vi "main.vi"() -> ()   [LabVIEW 2020]
uses:
  subVI/MsgBox.vi
  VarGLO/Global PEAK.vi
  <vilib>/regexp/Match Regular Expression.xnode
  VarGLO/Global var.vi
  VarGLO/VG_progressBar.vi
  f93c6fe3-7432-4718-be07-8f34c047d79f.vi
  VarGLO/Global PREDCIR.vi
  VarGLO/Global POSTDCIR.vi
  VarGLO/Global INTRADCIR.vi
  subVI/Ctrl/L2T.ctl
  <userlib>/Sylvain.lib/SN_type.ctl
panel:
  in  "TL?":bool
  in  "TypeVDA":T1
  out "POSTDCIR":T2
  out "PREDCIR":T2
  in  "40:2$ ok?":bool
  out "RunDCIR":bool
  out "INTRADCIR":T2
  out "dcir":string
  out "postdcir":string
  out "Numeric":i32 format="%.0f %"
  out "SNDCIR":string
  out "error out 2":errorcluster
  out "DCIR":u8(slide) scale=0.0..100.0
  in  "OFGETSVP$R":bool
  in  "stopask":bool
  in  "visadebug":refnum<visa-resource-name>
  out "String":string
  out "toute l'expression":string
  out "chaîne concaténée":string
  in  "image":string
  out "errout":errorcluster caption="sortie d'erreur"
  out "Image 2D":picture
  out "OFEnC":string caption="OF en cours coté Automate"
  out "err2":errorcluster
  out "MB":string
  in  "ValOFNext":bool
  in  "ok dem":bool
  in  "ValOF":bool
  out "intrafinal":string
  out "tableau ajouté":bool[](array[boolean])
  out "données":string[](array[string])
  out "OCV":string
  out "iso-":string
  out "iso+":string
  out "acir":string
  out "run..":i32(slide) scale=0.0..1000.0
  out "PN":string
  out "étage":string
  out "debug":T3
  in  "SimAuto":string caption="Simulateur automate"
  out "Check Final":bool
  out "mouchard OCV":string
  out "error out":errorcluster caption="Message erreur"
  in  "EXIT":bool
  out "L2T":T4 caption="Limites de test pris en compte"
  in  "OFnext":string caption="OF que l'on souhaite faire"
  out "STOP":bool
  out "Wdog":bool
  # "V3.3.0"
  # "Hors production\nZone de mise au point logiciel"
  # "Hors production\nZone de mise au point logiciel"
  # "--  Mouchard vers Auto  --"
  # "Test de mise au point"
  # "Pre DCIR_____________________________________"
  # "intra DCIR_____________________________________"
  # "Post DCIR_____________________________________"
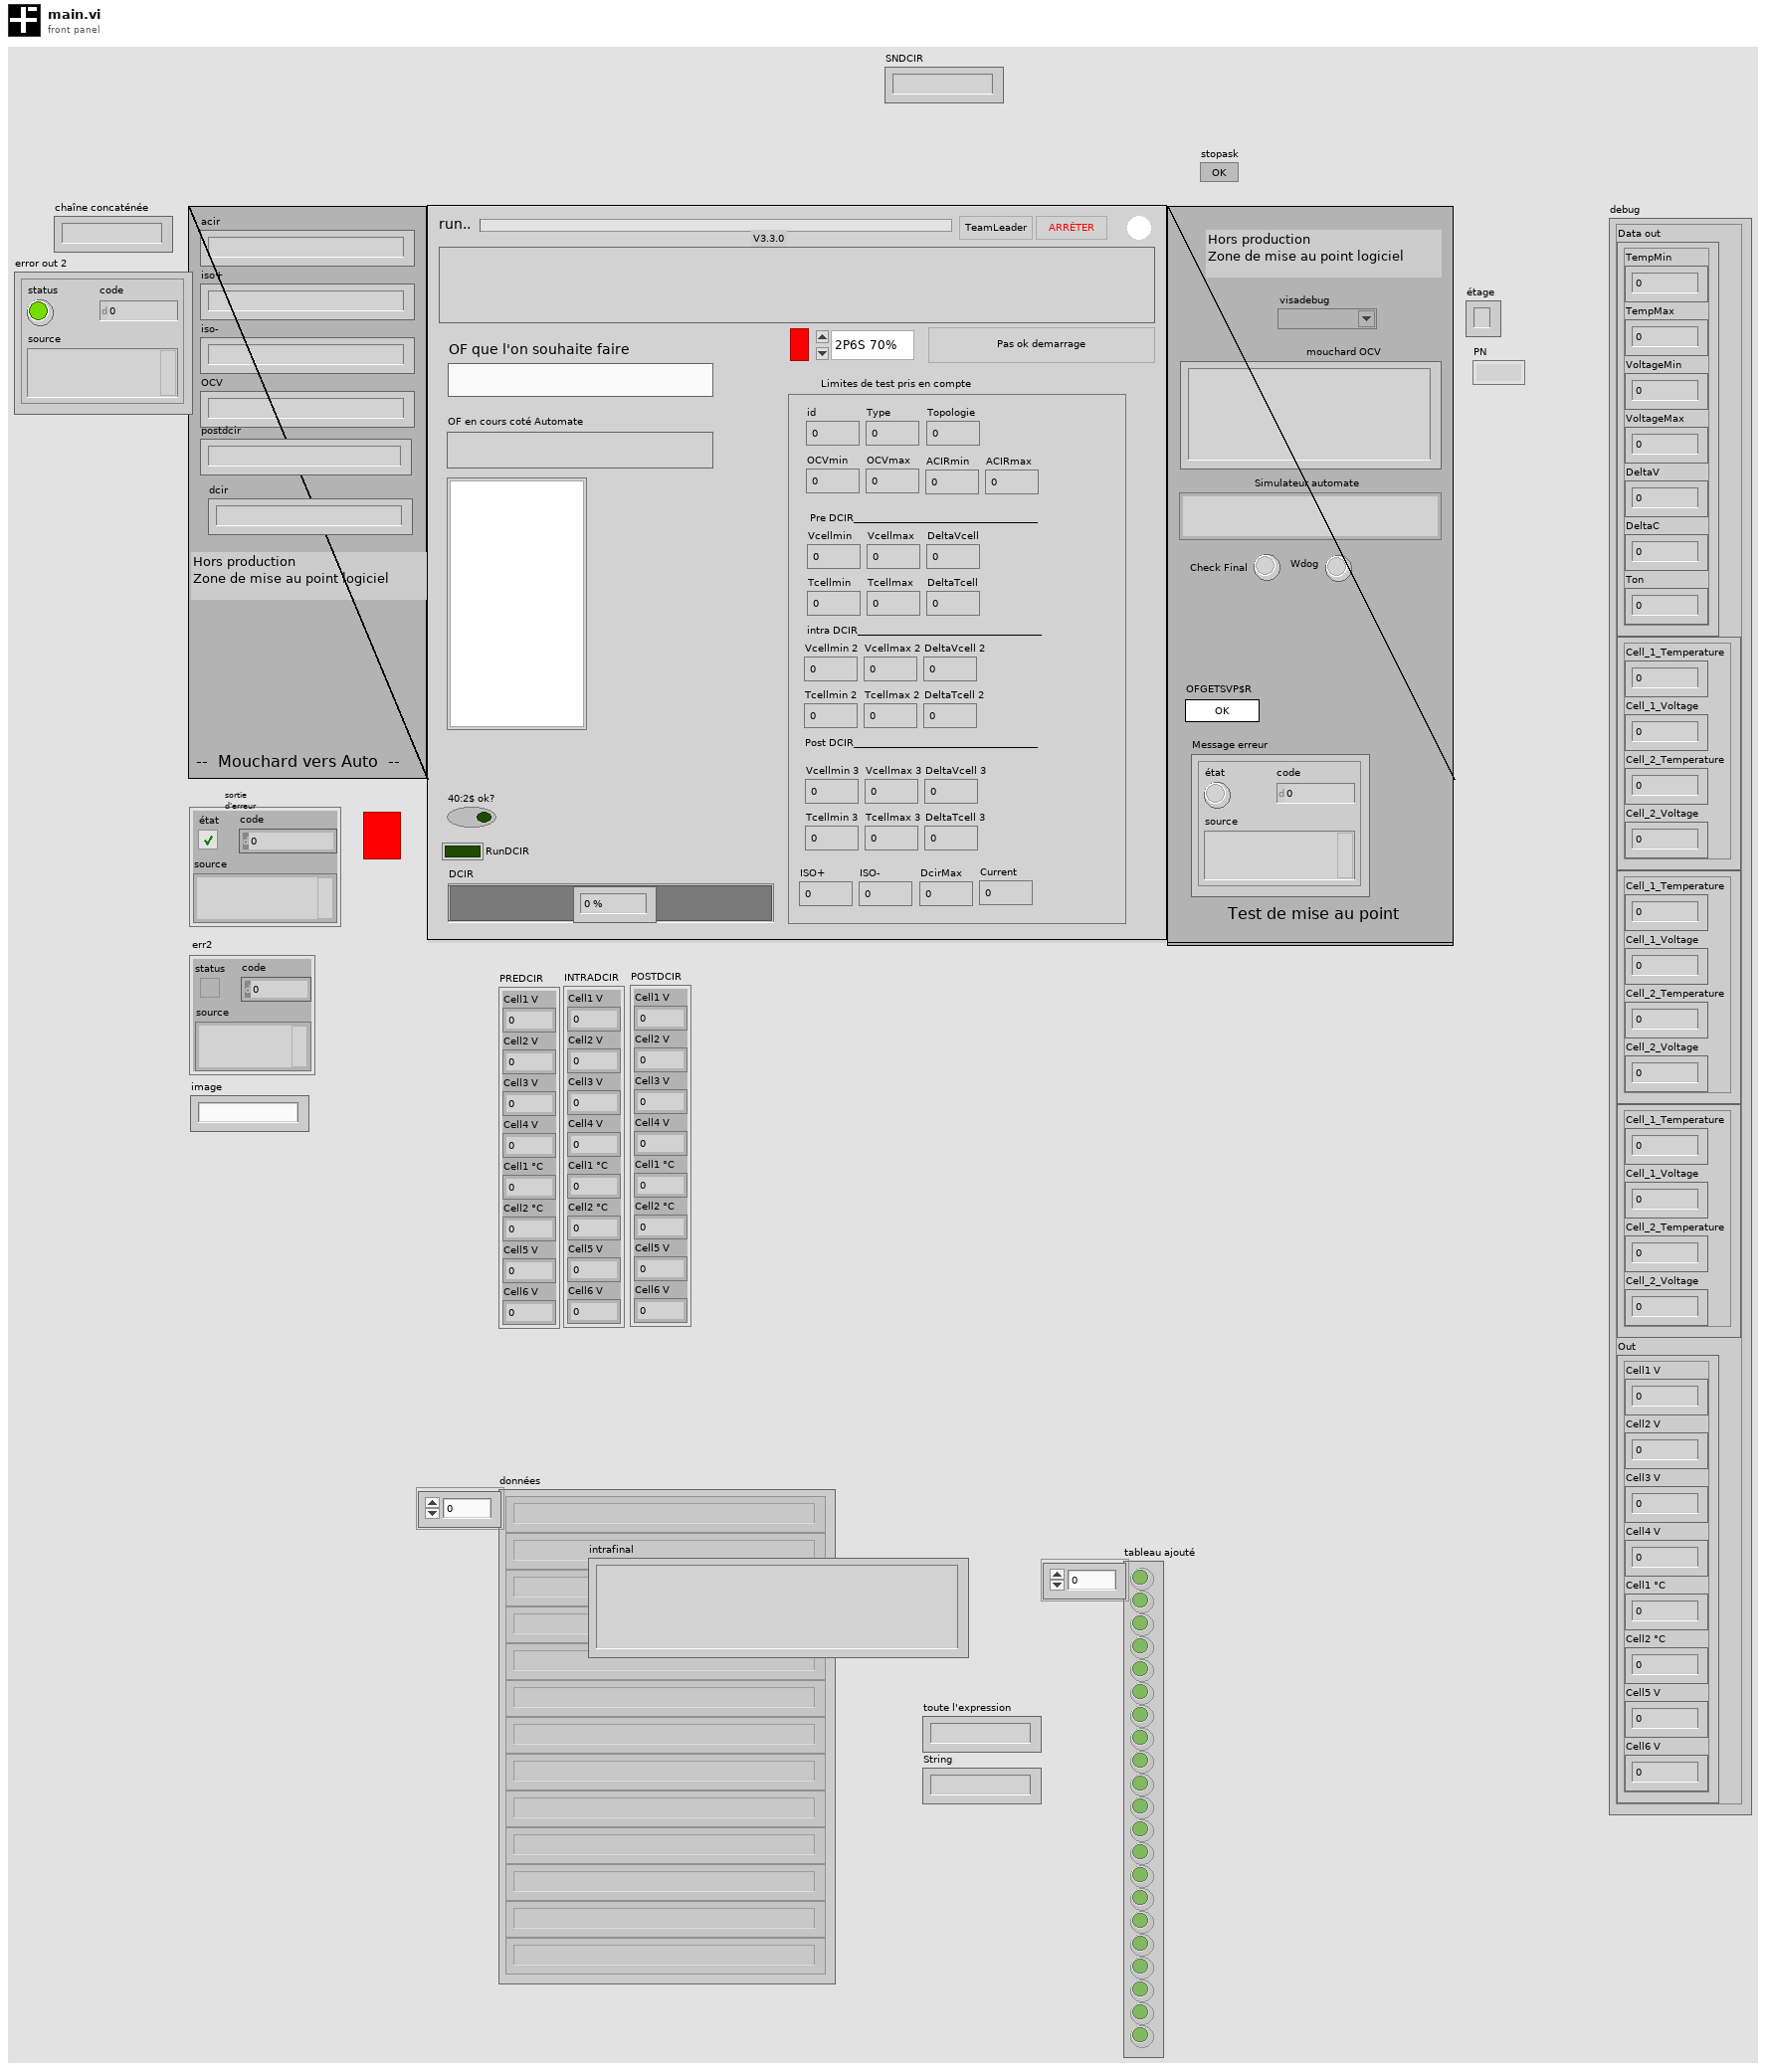
[diagram p1: front panel]
types:
  T1 = typedef "SN_type.ctl" = enum16{"2P6S 70%", "2P6S 30%", "3P4S 70%", "3P4S 30%"}
  T2 = cluster{"Cell1 V":sgl, "Cell2 V":sgl, "Cell3 V":sgl, "Cell4 V":sgl, "Cell1 °C":sgl, "Cell2 °C":sgl, "Cell5 V":sgl, "Cell6 V":sgl}
  T3 = cluster{"Data out":cluster{"TempMin":sgl, "TempMax":sgl, "VoltageMin":sgl, "VoltageMax":sgl, "DeltaV":sgl, "DeltaC":sgl, "Ton":sgl}, "Cluster":cluster{"Cell_1_Temperature":sgl, "Cell_1_Voltage":sgl, "Cell_2_Temperature":sgl, "Cell_2_Voltage":sgl}, "Cluster":cluster{"Cell_1_Temperature":sgl, "Cell_1_Voltage":sgl, "Cell_2_Temperature":sgl, "Cell_2_Voltage":sgl}, "Cluster":cluster{"Cell_1_Temperature":sgl, "Cell_1_Voltage":sgl, "Cell_2_Temperature":sgl, "Cell_2_Voltage":sgl}, "Out":cluster{"Cell1 V":sgl, "Cell2 V":sgl, "Cell3 V":sgl, "Cell4 V":sgl, "Cell1 °C":sgl, "Cell2 °C":sgl, "Cell5 V":sgl, "Cell6 V":sgl}}
  T4 = typedef "L2T.ctl" = cluster{"id":dbl, "Type":dbl, "OCVmin":dbl, "OCVmax":dbl, "ACIRmin":dbl, "ACIRmax":dbl, "Vcellmin":dbl, "Vcellmax":dbl, "DeltaVcell":dbl, "Tcellmin":dbl, "Tcellmax":dbl, "DeltaTcell":dbl, "ISO+":dbl, "ISO-":dbl, "DcirMax":dbl, "Current":dbl, "Topologie":dbl, "Vcellmin 2":dbl, "Vcellmax 2":dbl, "DeltaVcell 2":dbl, "Tcellmin 2":dbl, "Tcellmax 2":dbl, "DeltaTcell 2":dbl, "Vcellmin 3":dbl, "Vcellmax 3":dbl, "DeltaVcell 3":dbl, "Tcellmin 3":dbl, "Tcellmax 3":dbl, "DeltaTcell 3":dbl}
  T5 = cluster{"id":dbl, "Type":dbl, "OCVmin":dbl, "OCVmax":dbl, "ACIRmin":dbl, "ACIRmax":dbl, "Vcellmin":dbl, "Vcellmax":dbl, "DeltaVcell":dbl, "Tcellmin":dbl, "Tcellmax":dbl, "DeltaTcell":dbl, "ISO+":dbl, "ISO-":dbl, "DcirMax":dbl, "Current":dbl, "Topologie":dbl, "Vcellmin 2":dbl, "Vcellmax 2":dbl, "DeltaVcell 2":dbl, "Tcellmin 2":dbl, "Tcellmax 2":dbl, "DeltaTcell 2":dbl, "Vcellmin 3":dbl, "Vcellmax 3":dbl, "DeltaVcell 3":dbl, "Tcellmin 3":dbl, "Tcellmax 3":dbl, "DeltaTcell 3":dbl}
  T6 = typedef "PCANBasic.lvlib/Channel.ctl" = enum16{"PCAN_NONEBUS", "not used1", "not used2", "not used3", "not used4", "not used5", "not used6", "not used7", "not used8", "not used9", "not used10", "not used11", "not used12", "not used13", "not used14", "not used15", "not used16", "not used17", "not used18", "not used19", "not used20", "not used21", "not used22", "not used23", "not used24", "not used25", "not used26", "not used27", "not used28", "not used29", "not used30", "not used31", "not used32", "PCAN_ISABUS1", "PCAN_ISABUS2", "PCAN_ISABUS3", "PCAN_ISABUS4", "PCAN_ISABUS5", "PCAN_ISABUS6", "PCAN_ISABUS7", "PCAN_ISABUS8", "not used41", "not used42", "not used43", "not used44", "not used45", "not used46", "not used47", "not used48", "PCAN_DNGBUS1", "not used50", "not used51", "not used52", "not used53", "not used54", "not used55", "not used56", "not used57", "not used58", "not used59", "not used60", "not used61", "not used62", "not used63", "not used64", "PCAN_PCIBUS1", "PCAN_PCIBUS2", "PCAN_PCIBUS3", "PCAN_PCIBUS4", "PCAN_PCIBUS5", "PCAN_PCIBUS6", "PCAN_PCIBUS7", "PCAN_PCIBUS8", "not used73", "not used74", "not used75", "not used76", "not used77", "not used78", "not used79", "not used80", "PCAN_USBBUS1", "PCAN_USBBUS2", "PCAN_USBBUS3", "PCAN_USBBUS4", "PCAN_USBBUS5", "PCAN_USBBUS6", "PCAN_USBBUS7", "PCAN_USBBUS8", "Not used89", "Not used90", "Not used91", "Not used92", "Not used93", "Not used94", "Not used95", "Not used96", "PCAN_PCCBUS1", "PCAN_PCCBUS2"}
  T7 = typedef "imagedata.ctl" = cluster{"image type":i32, "image depth":i32, "image":u8[], "mask":u8[], "colors":u32[], "Rectangle":cluster{"left":i16, "top":i16, "right":i16, "bottom":i16}}
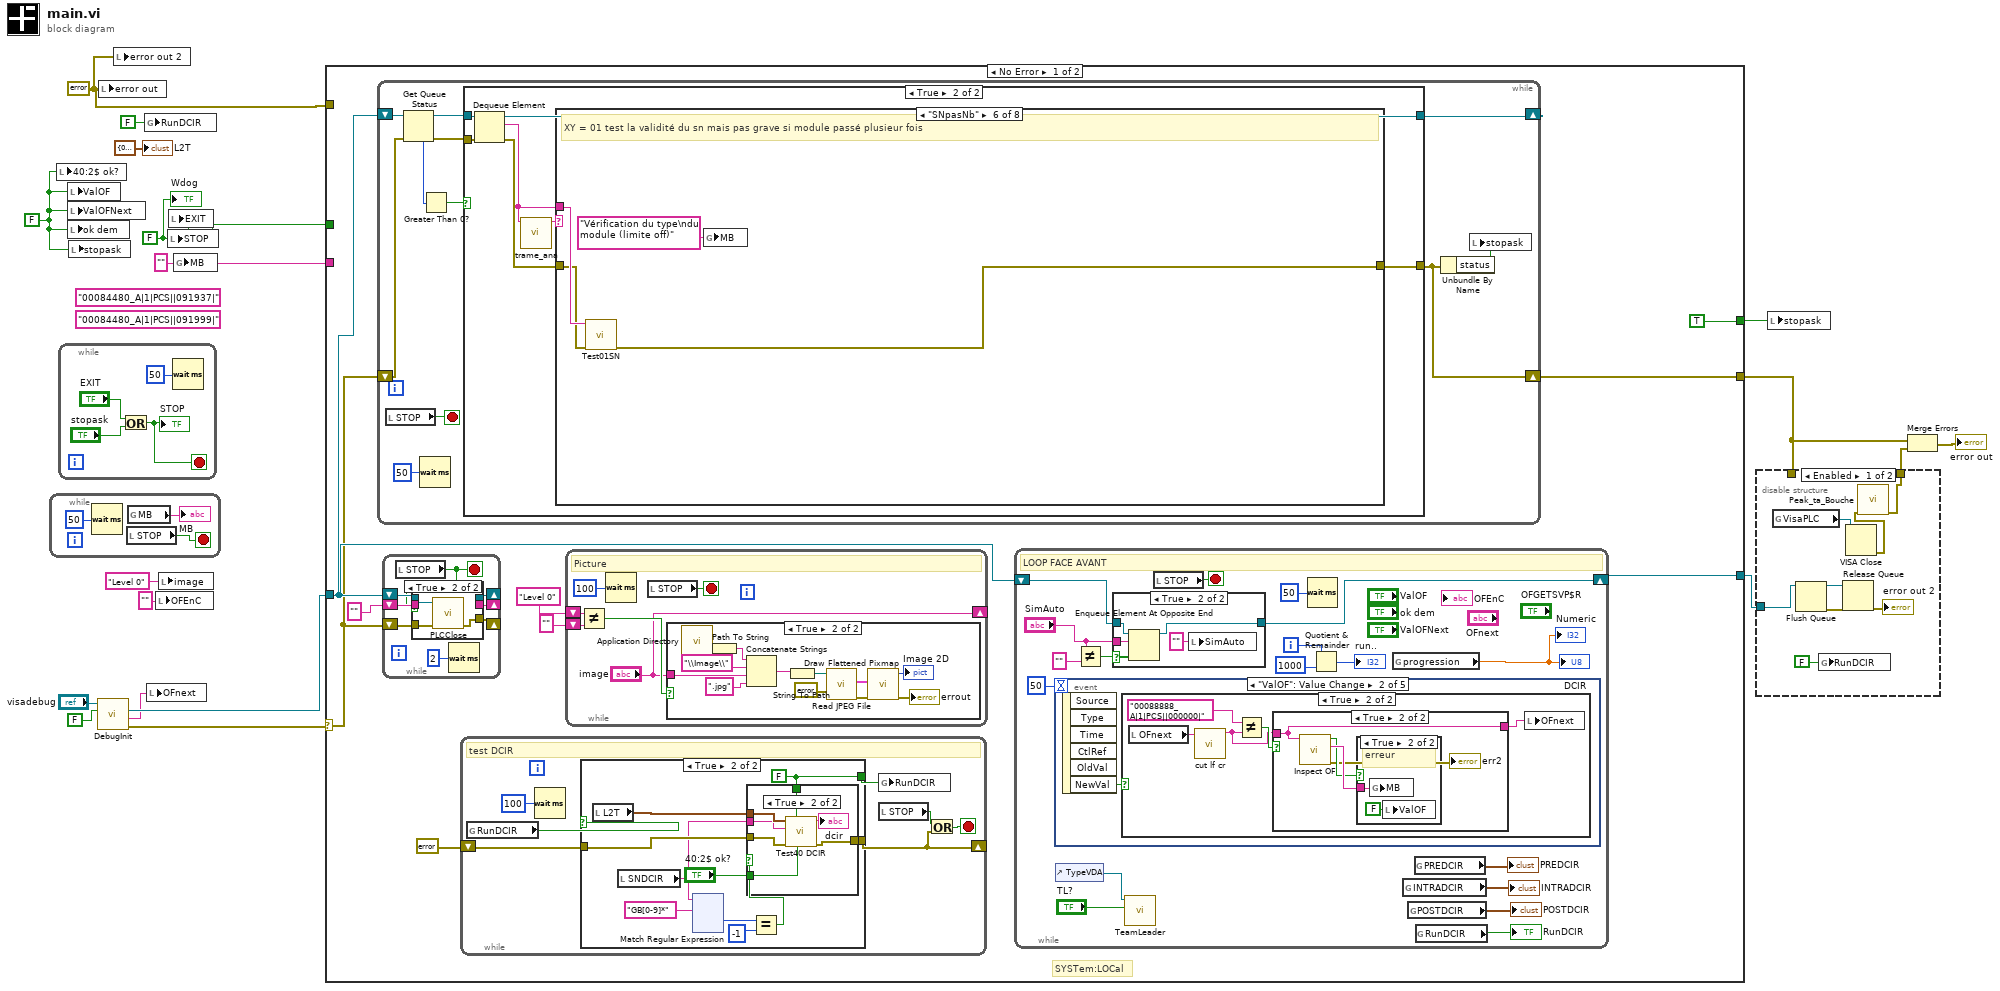
[diagram p0: block diagram]
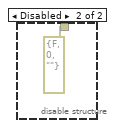
[diagram p2: hidden frame]
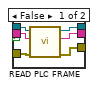
[diagram p3: hidden frame]
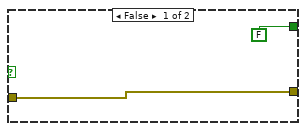
[diagram p4: hidden frame]
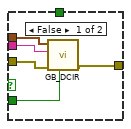
[diagram p5: hidden frame]
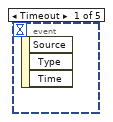
[diagram p6: hidden frame]
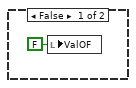
[diagram p7: hidden frame]
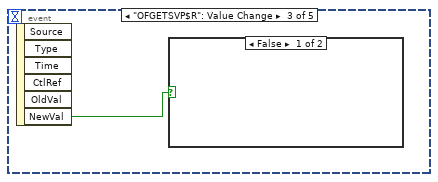
[diagram p10: hidden frame]
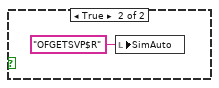
[diagram p11: hidden frame]
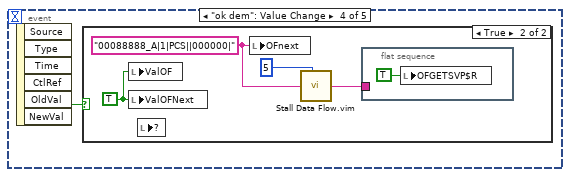
[diagram p12: hidden frame]
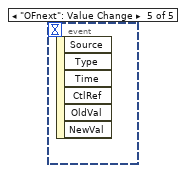
[diagram p14: hidden frame]
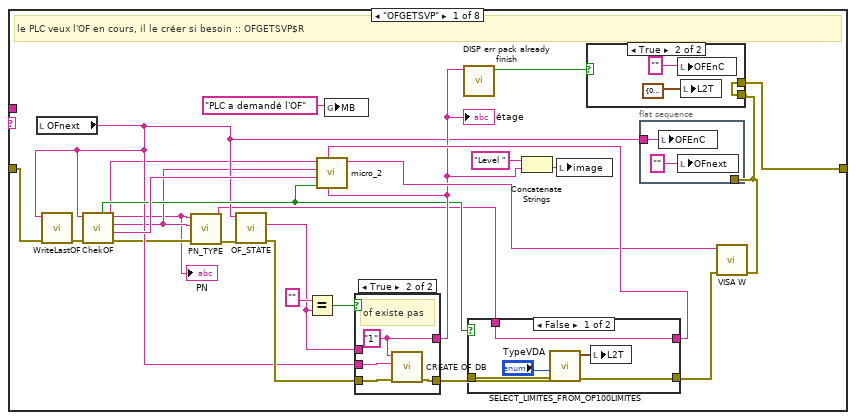
[diagram p17: hidden frame]
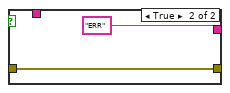
[diagram p20: hidden frame]
diagram:
  w1 = FALSE ("OF OK démarrage")
  w2 = errorcluster {"status"=FALSE, "code"=0, "source"=""} ("error out")
  (unwired) "00084480_A|1|PCS||091999|" ("OF à faire après")
  (unwired) "00084480_A|1|PCS||091937|" ("OF à faire")
  w14 = "" ("MSG")
  w18 = FALSE ("Tickwatchdog")
  n1 = while {
    stop <- w20 stop-if-true
    n2 = Wait (ms) ("Attendre (ms)")(milliseconds to wait=u32 50 ("attente (ms)")) -> ()  [unwired: 1 out]
    n3 = local read "STOP"() -> (w20:bool)
    n4 = global read "MsgBox.vi" "MB"() -> (→"MB":string)
  }
  n5 = local write "40:2$ ok?"(w1) -> ()
  n6 = while {
    stop <- w22 stop-if-true
    n7 = Or(x="EXIT", y="stopask") -> (x .or. y?=w22:bool)
    "STOP" <- w22
    n8 = Wait (ms)(milliseconds to wait=u32 50) -> ()  [unwired: 1 out]
  }
  n9 = local write "ValOF"(w1) -> ()
  n10 = local write "ValOFNext"(w1) -> ()
  n11 = local write "ok dem"(w1) -> ()
  n12 = local write "stopask"(w1) -> ()
  n13 = call "DebugInit.vi"("debug?"=FALSE ("s"), "VISA Refnum in"="visadebug") -> ("error out"=w10:errorcluster, "OF"=w11:string, "queue out"=w17:refnum<queue>)  [unwired: 7 in]
  n14 = local write "error out"(w2) -> ()
  n15 = local write "error out 2"(w2) -> ()
  n16 = global write "Global var.vi" "RunDCIR"(FALSE ("RunDCIR")) -> ()
  n17 = local write "OFnext"(w11) -> ()
  n18 = local write "OFEnC"("" ("OFEnC")) -> ()
  n19 = local write "image"("Level 0" ("image")) -> ()
  n20 = local write "STOP"(w18) -> ()
  n21 = local write "EXIT"(w18) -> ()
  n22 = global write "MsgBox.vi" "MB"(w14) -> ()
  n23 = case shown="No Error" w10 {
    selector: w10 -> [w29 w541]
    tunnel: w18 -> [_ _]
    tunnel: w14 -> [_ _]
    tunnel: w17 -> [w33 w539]
    tunnel: w2 -> [_ w544]
    tunnel: [w32 w544] -> w7
    tunnel: [TRUE TRUE] -> w5
    tunnel: [w27 w539] -> w4
    frame No Error {
      # "SYSTem:LOCal"
      n24 = while {
        shift-right: [w244] -> w32
        shift-left: w29 -> [w252]
        shift-right: [w248] -> _
        shift-left: w33 -> [w251]
        stop <- w246 stop-if-true
        n25 = local read "STOP"() -> (w246:bool)
        n26 = Get Queue Status ("Obtenir l'état d'une file d'attente")(queue=w251, error in (no error)=w252) -> (queue out=w250:refnum<queue>, error out=w249:errorcluster, # elements in queue=w245:i32)  [unwired: 1 in, 5 out]
        n27 = Wait (ms) ("Attendre (ms)")(milliseconds to wait=u32 50 ("attente (ms)")) -> ()  [unwired: 1 out]
        n28 = Greater Than 0?(x=w245) -> (x > 0?=w247:bool)
        n29 = case shown="True" w247 {
          tunnel: w250 -> [w253 w260]
          tunnel: w249 -> [w254 w259]
          tunnel: [w254 w257] -> w244
          tunnel: [w253 w256] -> w248
          frame False {
          }
          frame True {
            n30 = Dequeue Element(queue=w260, error in (no error)=w259) -> (queue out=w256:refnum<queue>, element=w255:string, error out=w258:errorcluster)  [unwired: 1 in, 1 out]
            n31 = call "trame_ana.vi"("Chaîne"=w255) -> ("Instruction"=w261:string)  [unwired: 10 in]
            n32 = case shown="\"SNpasNb\"" w261 {
              tunnel: w258 -> [w279 w309 w322 w495 w504 w512 w515 w520]
              tunnel: [w271 w308 w323 w494 w499 w514 w517 w520] -> w257
              tunnel: w255 -> [_ w312 w318 w492 w503 w513 w516 w519]
              frame "OFGETSVP" {
                # "le PLC veux l'OF en cours, il le créer si besoin :: OFGETSVP$R"
                n33 = local read "OFnext"() -> (w267:string)
                n34 = call "WriteLastOF.vi"("errin"=w279, "OF to save"=w267) -> ("errout"=w278:errorcluster)  [unwired: 9 in]
                n35 = call "ChekOF.vi"("errin"=w278, "OF in"=w267) -> ("errout"=w266:errorcluster, "SN"=w286:string, "version"=w265:string, "PN"=w264:string, "ArrsurErr"=w270:bool)  [unwired: 4 in, 1 out]
                "PN" <- w264
                n36 = call <userlib>:"PN_TYPE.vi"("errin"=w266, "Variante"=w265, "PN"=w264) -> ("errout"=w263:errorcluster, "element"=w262:string)  [unwired: 7 in]
                n37 = call <userlib>:"OF_STATE.vi"("errin"=w263, "OF"=w267) -> ("error out"=w269:errorcluster, "state str"=w268:string)  [unwired: 6 in, 2 out]
                n38 = Equal? ("Égaux ?")(x="", y=w268) -> (x = y?=w285:bool)
                n39 = global write "MsgBox.vi" "MB"("PLC a demandé l'OF" ("MSG")) -> ()
                n40 = case shown="True" w285 {
                  tunnel: w269 -> [w293 w298]
                  tunnel: w267 -> [_ w297]
                  tunnel: [w294 w296] -> w274
                  tunnel: w268 -> [w294 _]
                  tunnel: [w293 w295] -> w284
                  frame False {
                  }
                  frame True {
                    w296 = "1" ("result")
                    # "of existe pas"
                    n41 = call "CREATE OF DB.vi"("errin"=w298, "OF"=w297, "state"=w296) -> ("error out"=w295:errorcluster)  [unwired: 8 in]
                  }
                }
                "étage" <- w274
                n42 = call "DISP err pack already finish.vi"("result"=w274) -> ("étage3"=w273:bool)  [unwired: 10 in]
                n43 = case shown="False" w270 {
                  tunnel: [w303 w304] -> w283
                  tunnel: [w300 "ERR" ("Type")] -> w282
                  tunnel: w284 -> [w302 w304]
                  tunnel: w262 -> [w300 _]
                  frame False {
                    n44 = call <userlib>:"SELECT_LIMITES_FROM_OP100LIMITES.vi"("errin"=w302, "Enum"="TypeVDA") -> ("errout"=w303:errorcluster, "data"=w301:T4)  [unwired: 7 in, 1 out]
                    n45 = local write "L2T"(w301) -> ()
                  }
                  frame True {
                  }
                }
                n46 = call "micro_2.vi"("result"=w274, "Type"=w282, "err"=w270, "SN"=w286, "version"=w265, "PN"=w264) -> ("Chaîne"=w281:string)  [unwired: 5 in]
                n47 = Concatenate Strings("Level " ("string"), w274) -> (w275:string)
                n48 = local write "image"(w275) -> ()
                n49 = flat-sequence {
                  tunnel: w267 -> [w292]
                  tunnel: w272 -> [_]
                  frame #0 {
                    n50 = local write "OFEnC"(w292) -> ()
                    n51 = local write "OFnext"("" ("OFnext")) -> ()
                  }
                }
                n52 = call "VISA W.vi"("errin"=w283, "Chaîne"=w281) -> ("errout"=w272:errorcluster)  [unwired: 9 in]
                n53 = case shown="True" w273 {
                  tunnel: w272 -> [w287 w289]
                  tunnel: [w287 w289] -> w271
                  frame False {
                  }
                  frame True {
                    n54 = local write "OFEnC"("" ("OFEnC")) -> ()
                    n55 = local write "L2T"(T5 {"id"=0.0, "Type"=0.0, "OCVmin"=0.0, "OCVmax"=0.0, "ACIRmin"=0.0, "ACIRmax"=0.0, "Vcellmin"=0.0, "Vcellmax"=0.0, "DeltaVcell"=0.0, "Tcellmin"=0.0, "Tcellmax"=0.0, "DeltaTcell"=0.0, "ISO+"=0.0, "ISO-"=0.0, "DcirMax"=0.0, "Current"=0.0, "Topologie"=0.0, "Vcellmin 2"=0.0, "Vcellmax 2"=0.0, "DeltaVcell 2"=0.0, "Tcellmin 2"=0.0, "Tcellmax 2"=0.0, "DeltaTcell 2"=0.0, "Vcellmin 3"=0.0, "Vcellmax 3"=0.0, "DeltaVcell 3"=0.0, "Tcellmin 3"=0.0, "Tcellmax 3"=0.0, "DeltaTcell 3"=0.0} ("L2T")) -> ()
                  }
                }
              }
              frame "OFFINISH" {
                # "OFFINISHOK200084480_A|1|PCS||00001|$R"
                # "\" OFFINISHOK200084480_A|1|PCS||00001|$R \""
                n56 = local read "OFEnC"() -> (w310:string)
                n57 = local read "étage"() -> (w311:string)
                n58 = call "OFFINISH_compare.vi"("errin"=w309, "PlcFrame"=w312, "étage"=w311, "OFenC"=w310) -> ("errout"=w308:errorcluster, "OFEnC"=w306:string, "L2T"=w307:T5, "MB"=w313:string)  [unwired: 4 in]
                n59 = local write "OFEnC"(w306) -> ()
                n60 = global write "MsgBox.vi" "MB"(w313) -> ()
                n61 = local write "L2T"(w307) -> ()
              }
              frame "Requette" {
                # "SN"
                n62 = String Subset ("Sous-ensemble d'une chaîne")(string=w318, length (rest)=2 ("longueur (reste)")) -> (substring=w324:string)  [unwired: 1 in]
                n63 = xnode "Match Regular Expression"("chaîne en entrée"=w318, "expression régulière"="[0-9 A-Z]*:", "offset (0)"=2) -> ("toute l'expression"=w317:string, "après la correspondance"=w321:string)  [unwired: 3 in, 3 out]
                n64 = Search and Replace String ("Rechercher et remplacer une chaîne")(input string=w321, search string="$R" ("chaîne recherchée")) -> (result string=w319:string)  [unwired: 6 in, 3 out]
                n65 = Search and Replace String(input string=w317, search string=":", replace string="" ("replace string (\"\")")) -> (result string=w314:string)  [unwired: 5 in, 3 out]
                n66 = case shown="\"50\"" w324 {
                  tunnel: [w329 w339 w346 w352 w358 w364 w371] -> w323
                  tunnel: w322 -> [w329 w340 w343 w349 w355 w364 w373]
                  tunnel: w319 -> [_ w338 w347 w353 w361 _ _]
                  tunnel: w314 -> [_ w336 w345 w351 w360 w362 w370]
                  frame "Faux", Default {
                    n67 = global write "MsgBox.vi" "MB"("J'ai recu une trame non comprise" ("MSG")) -> ()
                  }
                  frame "10" {
                    w337 = "!!!!!" ("chaîne")
                    # "OCV ( PLC ) + CMODpredcir( PC )"
                    n68 = local read "L2T"() -> (w330:T4)
                    n69 = global read "Global PEAK.vi" "T10"() -> (w331:T6)
                    n70 = global write "MsgBox.vi" "MB"("PLC demande à verifier\nl'OCV" ("MSG")) -> ()
                    n71 = call "Test10.vi"("Peak"=w331, "L2T"=w330, "errin"=w340, "SN"=w336, "OCV"=w338) -> ("errout"=w339:errorcluster, "chaîne concaténée"=w335:string, "cluster de sortie"=→"debug":T3)  [unwired: 3 in, 1 out]
                    n72 = Concatenate Strings(w338, w337, w336, w337, w335) -> (→"mouchard OCV":string)
                  }
                  frame "11" {
                    # "ACIR :: PLC"
                    n73 = local read "L2T"() -> (w341:T4)
                    n74 = call "Test11ACiR.vi"("errin"=w343, "L2T 2"=w341, "result string"=w347, "SN"=w345) -> ("error out"=w346:errorcluster, "String"=→"acir":string)  [unwired: 6 in]
                    n75 = global write "MsgBox.vi" "MB"("Le PLC demande à verifier \nl'ACIR" ("MSG")) -> ()
                  }
                  frame "20" {
                    # "ISOLEMENT BAT + :: PLC"
                    n76 = local read "L2T"() -> (w354:T4)
                    n77 = call "Test20ISO+.vi"("errin"=w349, "L2T 2"=w354, "mesure"=w353, "SN"=w351) -> ("error out"=w352:errorcluster, "iso+"=→"iso+":string)  [unwired: 6 in]
                    n78 = global write "MsgBox.vi" "MB"("Le PLC veux vérifier\nl'isolement BAT+" ("MSG")) -> ()
                  }
                  frame "30" {
                    # "ISOLEMENT BAT -  :: PLC"
                    n79 = local read "L2T"() -> (w359:T4)
                    n80 = call "Test30ISOmoins.vi"("errin"=w355, "L2T"=w359, "Value"=w361, "SN"=w360) -> ("error out"=w358:errorcluster, "ISO-"=→"iso-":string)  [unwired: 6 in]
                    n81 = global write "MsgBox.vi" "MB"("Le PLC veux vérifier\nl'isolement BAT-" ("MSG")) -> ()
                  }
                  frame "40" {
                    # "400B5MEVA000CA1JC1M5525088:0$R"
                    # "DCIR :: PC"
                    n82 = global write "Global var.vi" "RunDCIR"(TRUE) -> ()
                    n83 = global write "MsgBox.vi" "MB"("PLC demande un DCIR" ("MSG")) -> ()
                    "SNDCIR" <- w362
                  }
                  frame "50" {
                    # "post DCIR :: PC"
                    n84 = global read "Global PEAK.vi" "T50"() -> (w374:T6)
                    n85 = local read "L2T"() -> (w367:T4)
                    n86 = call "Test50.vi"("L2T"=w367, "SN"=w370, "errin"=w373, "Peak"=w374) -> ("v1"=→"postdcir":string, "errout"=w372:errorcluster)  [unwired: 4 in, 1 out]
                    n87 = call "FinalCheck.vi"("errin"=w372, "L2T"=w367, "SN"=w370) -> ("error out"=w371:errorcluster, "ET logique"=→"Check Final":bool)  [unwired: 4 in, 3 out]
                    n88 = global write "MsgBox.vi" "MB"("PLC demande un Post DCIR" ("MSG")) -> ()
                  }
                }
              }
              frame "TracaHIOKI" {
                # "INSERT INTO `zen+`.`op100eqsn` (`id`, `PNvers`, `etageencours`, `snst5520isoplus`\n, `snst5520isomoins`, `snbt3563`, `date`) VALUES ('3', 'OFIII', '2', 'iso+', 'iso-', '35', '2023-06-06 23:55:33');"
                n89 = local read "étage"() -> (w491:string)
                n90 = local read "PN"() -> (w490:string)
                n91 = call "TracaHioki.vi"("errin"=w495, "datain"=w492, "etage"=w491, "PN"=w490) -> ("error out"=w494:errorcluster, "out"=w493:string)  [unwired: 6 in]
                n92 = local write "mouchard OCV"(w493) -> ()
                n93 = global write "MsgBox.vi" "MB"("Je releve le SN du ST5520 Iso+" ("Message BOX")) -> ()
              }
              frame "SN" {
                # "XY = 00 test la validité du SN"
                n94 = local read "L2T"() -> (w496:T4)
                n95 = call "Test00SN.vi"("errin"=w504, "L2T 2"=w496, "String in"=w503) -> ("errout"=w500:errorcluster, "toute l'expression"=w502:string, "Boolean"=w498:bool, "String out"=w501:string)  [unwired: 5 in]
                n96 = case shown="True" w498 {
                  tunnel: w502 -> [_ w510]
                  tunnel: w501 -> [_ w509]
                  tunnel: w500 -> [w505 w508]
                  tunnel: [w505 w507] -> w499
                  frame False {
                  }
                  frame True {
                    n97 = call "Init Data BDD.vi"("errin"=w508, "Type"=w509, "SN"=w510) -> ("error out"=w507:errorcluster, "chaîne concaténée"=→"chaîne concaténée":string)  [unwired: 7 in]
                    "toute l'expression" <- w510
                    "String" <- w509
                  }
                }
                n98 = global write "MsgBox.vi" "MB"("Vérification du SN et du type\ndu module" ("Message BOX")) -> ()
              }
              frame "SNpasNb" {
                # "XY = 01 test la validité du sn mais pas grave si module passé plusieur fois"
                n99 = call "Test01SN.vi"("errin"=w512, "String"=w513) -> ("errout"=w514:errorcluster)  [unwired: 9 in]
                n100 = global write "MsgBox.vi" "MB"("Vérification du type\ndu module (limite off)" ("Message BOX")) -> ()
              }
              frame "GB" {
                # "Cas des Goldens boards Obsolète"
                n101 = call "TestGB.vi"("errin"=w515, "String"=w516) -> ("errout"=w517:errorcluster)  [unwired: 9 in]
                n102 = global write "MsgBox.vi" "MB"("Golden Board engagé" ("Message BOX")) -> ()
              }
              frame "ERR", Default {
                n103 = call "DISP err unknow request.vi"("String"=w519) -> ()  [unwired: 11 in]
              }
            }
          }
        }
        n104 = Unbundle By Name(w244) -> ("status"=w243:bool)
        n105 = local write "stopask"(w243) -> ()
      }
      n106 = while {
        shift-right: [w37] -> _
        shift-left: "" -> [w38]
        shift-right: [w39] -> _
        shift-left: w29 -> [w42]
        shift-right: [w40] -> _
        shift-left: w33 -> [w41]
        stop <- w36 stop-if-true
        n107 = local read "STOP"() -> (w36:bool)
        n108 = case shown="True" w36 {
          tunnel: w42 -> [w48 w51]
          tunnel: w41 -> [w47 w50]
          tunnel: [w46 _] -> w40
          tunnel: [w45 w49] -> w39
          tunnel: w38 -> [w44 _]
          tunnel: [w43 _] -> w37
          frame False {
            n109 = call "READ PLC FRAME.vi"("errin"=w48, "String in"=w44, "Queue in"=w47) -> ("errout"=w45:errorcluster, "String out"=w43:string, "Queue out"=w46:refnum<queue>)  [unwired: 6 in]
          }
          frame True {
            n110 = call "PLCClose.vi"("error in (no error)"=w51, "Queue in"=w50) -> ("error out"=w49:errorcluster)  [unwired: 9 in]
          }
        }
        n111 = Wait (ms)(milliseconds to wait=u32 2) -> ()  [unwired: 1 out]
      }
      n112 = while {
        shift-right: [w55] -> _
        shift-left: errorcluster {"status"=FALSE, "code"=0, "source"=""} ("errout") -> [w56]
        stop <- w53 stop-if-true
        # "test DCIR"
        n113 = global read "Global var.vi" "RunDCIR"() -> (w57:bool)
        n114 = Wait (ms) ("Attendre (ms)")(milliseconds to wait=u32 100 ("attente (ms)")) -> ()  [unwired: 1 out]
        n115 = case shown="True" w57 {
          tunnel: w56 -> [w60 w69]
          tunnel: [w60 w68] -> w55
          tunnel: [FALSE ("3P4S") w67] -> w52
          frame False {
          }
          frame True {
            w67 = FALSE ("3P4S")
            n116 = local read "L2T"() -> (w70:T4)
            n117 = local read "SNDCIR"() -> (w65:string)
            n118 = xnode "Match Regular Expression"("input string"=w65, "regular expression"="GB[0-9]*") -> ("offset past match"=w64:i32)  [unwired: 4 in, 4 out]
            n119 = Equal?(x=w64, y=-1) -> (x = y?=w62:bool)
            n120 = case shown="True" w62 {
              tunnel: w70 -> [w72 w82]
              tunnel: w69 -> [w74 w81]
              tunnel: [w75 w80] -> w68
              tunnel: w67 -> [_ w79]
              tunnel: w65 -> [w73 w78]
              tunnel: "40:2$ ok?" -> [w71 w76]
              frame False {
                n121 = call "GB_DCIR.vi"("40:2$ ok?"=w71, "errin"=w74, "SN"=w73, "L2T 2"=w72) -> ("errout"=w75:errorcluster)  [unwired: 7 in]
              }
              frame True {
                n122 = call "Test40 DCIR.vi"("40:2$ ok?"=w76, "3P4S"=w79, "errin"=w81, "SN"=w78, "L2T 2"=w82) -> ("errout"=w80:errorcluster, "v1"=→"dcir":string)  [unwired: 1 in, 4 out]
              }
            }
          }
        }
        n123 = global write "Global var.vi" "RunDCIR"(w52) -> ()
        n124 = local read "STOP"() -> (w54:bool)
        n125 = Or(x=w54, y=w55) -> (x .or. y?=w53:bool)
      }
      n126 = while {
        shift-right: ["image"] -> _
        shift-left: "" ("image") -> [w522]
        shift-left: "Level 0" ("image") -> [w521]
        stop <- w525 stop-if-true
        # "Picture"
        n127 = Not Equal?(x=w521, y=w522) -> (x != y?=w524:bool)
        n128 = Wait (ms) ("Attendre (ms)")(milliseconds to wait=u32 100 ("attente (ms)")) -> ()  [unwired: 1 out]
        n129 = local read "STOP"() -> (w525:bool)
        n130 = case shown="True" w524 {
          tunnel: "image" -> [_ w536]
          frame False {
          }
          frame True {
            n131 = call <vilib>:"Application Directory.vi"() -> ("Application Directory"=w532:path)
            n132 = Path To String(path=w532) -> (string=w533:string)
            n133 = Concatenate Strings(w533, "\\Image\\" ("chaîne"), w536, ".jpg" ("chaîne")) -> (w531:string)
            n134 = String To Path(string=w531) -> (path=w530:path)
            n135 = call <vilib>:"Read JPEG File.vi"("error in (no error)"=errorcluster {"status"=FALSE, "code"=0, "source"=""}, "path to JPEG file"=w530) -> ("error out"=→"errout":errorcluster, "image data"=w537:T7)  [unwired: 7 in, 1 out]
            n136 = call <vilib>:"Draw Flattened Pixmap.vi"("image data"=w537) -> ("new picture"=→"Image 2D":picture)  [unwired: 8 in]
          }
        }
      }
      n137 = while {
        shift-right: [w211] -> w27
        shift-left: w33 -> [w212]
        i -> [w205]
        stop <- w214 stop-if-true
        # "LOOP FACE AVANT"
        n138 = event shown="[1] \"ValOF\": Value Change" {
          selector: _ -> [_ _ _ _ _]
          dyn-events: _ -> [_ _ _ _ _]
          timeout: 50 -> [_ _ _ _ _]
          event Timeout {
            n139 = event-data() -> ()  [unwired: 1 in, 3 out]
          }
          event "ValOF": Value Change {
            n140 = event-data() -> ("NewVal"=w215:bool)  [unwired: 1 in, 5 out]
            n141 = case shown="True" w215 {
              frame False {
                n142 = local write "ValOF"(FALSE ("Bouton Jouer")) -> ()
              }
              frame True {
                n143 = local read "OFnext"() -> (w221:string)
                n144 = call "cut lf cr.vi"("strin"=w221) -> ("strout"=w217:string)  [unwired: 10 in]
                n145 = Not Equal?(x="00088888_A|1|PCS||000000|", y=w217) -> (x != y?=w219:bool)
                n146 = case shown="True" w219 {
                  tunnel: w217 -> [w222 w223]
                  tunnel: [w222 w223] -> w218
                  frame False {
                  }
                  frame True {
                    n147 = call "Inspect OF.vi"("OF"=w223) -> ("error out"=→"err2":errorcluster, "cas faux"=w226:string, "Boolean"=w225:bool)  [unwired: 8 in]
                    n148 = case shown="True" w225 {
                      tunnel: w226 -> [_ w227]
                      frame False {
                      }
                      frame True {
                        # "erreur"
                        n149 = global write "MsgBox.vi" "MB"(w227) -> ()
                        n150 = local write "ValOF"(FALSE ("Bouton Jouer")) -> ()
                      }
                    }
                  }
                }
                n151 = local write "OFnext"(w218) -> ()
              }
            }
          }
          event "OFGETSVP$R": Value Change {
            n152 = event-data() -> ("NewVal"=w229:bool)  [unwired: 1 in, 5 out]
            n153 = case shown="False" w229 {
              frame False {
              }
              frame True {
                n154 = local write "SimAuto"("OFGETSVP$R" ("SimAuto")) -> ()
              }
            }
          }
          event "ok dem": Value Change {
            n155 = event-data() -> ("NewVal"=w231:bool)  [unwired: 1 in, 5 out]
            n156 = case shown="True" w231 {
              frame False {
              }
              frame True {
                w235 = TRUE ("Bouton Jouer")
                w234 = "00088888_A|1|PCS||000000|" ("OF à faire")
                n157 = local write "ValOF"(w235) -> ()
                n158 = local write "ValOFNext"(w235) -> ()
                n159 = local read item#-1() -> ()  [unwired: 1 in]
                n160 = local write "OFnext"(w234) -> ()
                n161 = call "Stall Data Flow.vim"("value in"=w234, "milliseconds to wait"=u32 5) -> ("value out"=w233:string)  [unwired: 1 out]
                n162 = flat-sequence {
                  tunnel: w233 -> [_]
                  frame #0 {
                    n163 = local write "OFGETSVP$R"(TRUE ("OFGETSVP$R")) -> ()
                  }
                }
              }
            }
          }
          event "OFnext": Value Change {
            n164 = event-data() -> ()  [unwired: 1 in, 6 out]
          }
        }
        n165 = control-ref of="TypeVDA"() -> (w198:refnum<vi>)
        n166 = Not Equal? ("Différents ?")(x="SimAuto", y="") -> (x != y?=w208:bool)
        n167 = case shown="True" w208 {
          tunnel: w212 -> [w237 w241]
          tunnel: [w237 w240] -> w211
          tunnel: "SimAuto" -> [_ w239]
          frame False {
          }
          frame True {
            n168 = Enqueue Element At Opposite End(queue=w241, element=w239) -> (queue out=w240:refnum<queue>)  [unwired: 2 in, 2 out]
            n169 = local write "SimAuto"("" ("PUTTY")) -> ()
          }
        }
        n170 = call "TeamLeader.vi"("TL?"="TL?", "Enum in"=w198) -> ()  [unwired: 10 in]
        n171 = local read "STOP"() -> (w214:bool)
        n172 = Wait (ms) ("Attendre (ms)")(milliseconds to wait=u32 50 ("attente (ms)")) -> ()  [unwired: 1 out]
        n173 = Quotient & Remainder ("Quotient et Reste")(x=w205, y=1000) -> (x-y*floor(x/y)=→"run..":i32)  [unwired: 1 out]
        n174 = global read "VG_progressBar.vi" "progression"() -> (→"DCIR" →"Numeric":dbl)
        n175 = global read "Global INTRADCIR.vi" "INTRADCIR"() -> (→"INTRADCIR":T2)
        n176 = global read "Global POSTDCIR.vi" "POSTDCIR"() -> (→"POSTDCIR":T2)
        n177 = global read "Global PREDCIR.vi" "PREDCIR"() -> (→"PREDCIR":T2)
        n178 = global read "Global var.vi" "RunDCIR"() -> (→"RunDCIR":bool)
      }
    }
    frame Error {
      n179 = Unbundle By Name(w541) -> ("source"=w546:string)
      n180 = global write "Global var.vi" "RunDCIR"(FALSE ("RunDCIR")) -> ()
      n181 = local write "STOP"(TRUE ("STOP")) -> ()
      n182 = Concatenate Strings("Err d'initialisation; \nDu peak can ou de la communication série" ("MSG"), "\r\n", w546) -> (w543:string)
      n183 = global write "MsgBox.vi" "MB"(w543) -> ()
    }
  }
  n184 = disable-structure shown="Enabled" {
    disable-tunnel: [w550 errorcluster {"status"=FALSE, "code"=0, "source"=""} ("sortie d'erreur")] -> w15
    disable-tunnel: w7 -> [_ _]
    disable-tunnel: w4 -> [w553 _]
    frame Enabled {
      n185 = global read "Global PEAK.vi" "VisaPLC"() -> (w554:refnum<visa-resource-name>)
      n186 = Flush Queue(queue=w553) -> (queue out=w552:refnum<queue>, error out=w551:errorcluster)  [unwired: 1 in, 1 out]
      n187 = global write "Global var.vi" "RunDCIR"(FALSE ("RunDCIR")) -> ()
      n188 = Release Queue(queue=w552, error in (no error)=w551) -> (error out=→"error out 2":errorcluster)  [unwired: 1 in, 2 out]
      n189 = VISA Close(VISA resource name=w554) -> (error out=w555:errorcluster)  [unwired: 1 in]
      n190 = call <userlib>:"Peak_ta_Bouche.vi"("errin"=w555) -> ("sortie d'erreur"=w550:errorcluster)  [unwired: 8 in, 2 out]
    }
    frame Disabled {
    }
  }
  n191 = local write "stopask"(w5) -> ()
  n192 = Merge Errors(w7, w15) -> (→"error out":errorcluster)
  "Wdog" <- w18
  "L2T" <- T5 {"id"=0.0, "Type"=0.0, "OCVmin"=0.0, "OCVmax"=0.0, "ACIRmin"=0.0, "ACIRmax"=0.0, "Vcellmin"=0.0, "Vcellmax"=0.0, "DeltaVcell"=0.0, "Tcellmin"=0.0, "Tcellmax"=0.0, "DeltaTcell"=0.0, "ISO+"=0.0, "ISO-"=0.0, "DcirMax"=0.0, "Current"=0.0, "Topologie"=0.0, "Vcellmin 2"=0.0, "Vcellmax 2"=0.0, "DeltaVcell 2"=0.0, "Tcellmin 2"=0.0, "Tcellmax 2"=0.0, "DeltaTcell 2"=0.0, "Vcellmin 3"=0.0, "Vcellmax 3"=0.0, "DeltaVcell 3"=0.0, "Tcellmin 3"=0.0, "Tcellmax 3"=0.0, "DeltaTcell 3"=0.0} ("L2T")
